vi "Lookup class.vi"(8 "error in":errorcluster, 10 "Class name":string) -> (0 "error out":errorcluster, 3 "Read Config out":refnum<class "Read Config File.lvclass">)   [LabVIEW 2025, in "Config Library.lvlib" / "Read Config File.lvclass"]
uses:
  Read Config File.lvclass
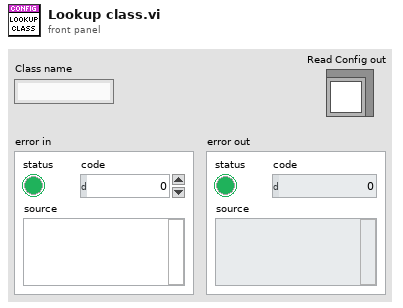
[diagram p1: front panel]
types:
  T1 = map{string, refnum<class "Read Config File.lvclass">}
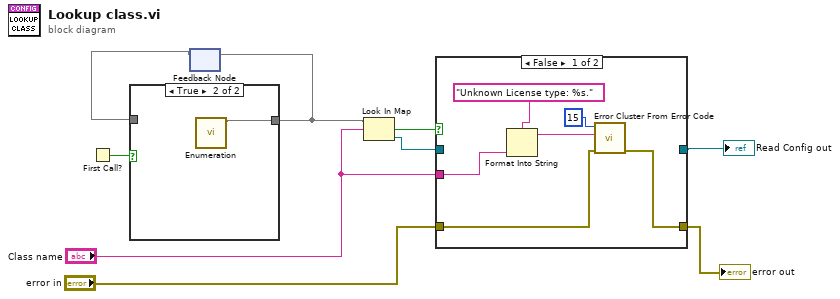
[diagram p0: block diagram]
diagram:
  n1 = First Call?() -> (First Call?: T/F=w9:bool)
  n2 = feedback #1() -> (w8:T1)  [unwired: 1 in]
  n3 = case shown="True" w9 {
    tunnel: w8 -> [w10 _]
    tunnel: [w10 w11] -> w7
    frame False {
    }
    frame True {
      n4 = call "Enumeration.vi"() -> ("Enumeration"=w11:T1)  [unwired: 11 in]
    }
  }
  n5 = feedback-in #1(w7) -> ()
  n6 = Look In Map(map=w7, key="Class name") -> (key not found?=w6:bool, value=w2:refnum<class "Read Config File.lvclass">)  [unwired: 1 in]
  n7 = case shown="False" w6 {
    tunnel: [w15 w19] -> w5
    tunnel: "error in" -> [w14 w19]
    tunnel: "Class name" -> [w12 _]
    tunnel: [_ w18] -> w1
    tunnel: w2 -> [_ w18]
    frame False {
      n8 = Format Into String(format string="Unknown License type: %s.", w12) -> (resulting string=w17:string)  [unwired: 2 in, 1 out]
      n9 = call <vilib>:"Error Cluster From Error Code.vi"("error in (no error)"=w14, "error message (\"\")"=w17, "error code (0)"=15) -> ("error out"=w15:errorcluster)  [unwired: 6 in]
    }
    frame True {
    }
  }
  "Read Config out" <- w1
  "error out" <- w5
